vi "3_Analog_Meter_Reader(Inference).vi"() -> ()   [LabVIEW 2020]
uses:
  <vilib>/Ngene/DeepLTK/Toolkit/NN_Network/Controls/NN_Save_Before_Destroy_Options.ctl
  <vilib>/Ngene/DeepLTK/Toolkit/NN_Layers/Layers/Input/API/NN_Layer_Set_Out(Input3D_idx).vi
  <vilib>/Ngene/DeepLTK/Toolkit/Deep_Learning_Toolkit_by_Ngene.lvlib
  <vilib>/vision/NI_Vision_Development_Module.lvlib
panel:
  out "Inference Speed (FPS)":dbl=427.1678770791453
  out "Image Path":path=path "D:/DeepLTK_Examples/Analog_Meter/Train/Images/0537.png"
  in  "Stop":bool
  out "Predictions":sgl[](array[slide])=[74.73664] scale=0.0..10.0
  in  "mBatch":i32=1
  in  "NN Device":enum16{"CPU", "GPU"}(ring)=enum."GPU"
  in  "Network Configuration File Path":path=path "D:/Ngene/GitHub/deepltk_examples/3_Image_Processing/31_Image_Regression/working/Analog_Meter/Analog_Meter_net_cfg_23_11_29__18_30_17.cfg"
  in  "Weight File Path":path=path "D:/Ngene/GitHub/deepltk_examples/3_Image_Processing/31_Image_Regression/working/Analog_Meter/Analog_Meter_weights_23_11_29__18_30_17.bin"
  in  "File Path":path=path "D:/DeepLTK_Examples/Analog_Meter/Train/Images/0537.png"
  out "Image":T1(plugin-control)
  # "Instructions:\n1. Provide model files (.cfg and .bin).\n2. Run the VI\n3. Drag and drop image on \"Input Image\"\n4. Observe rge prediction result."
  # "Input Image"
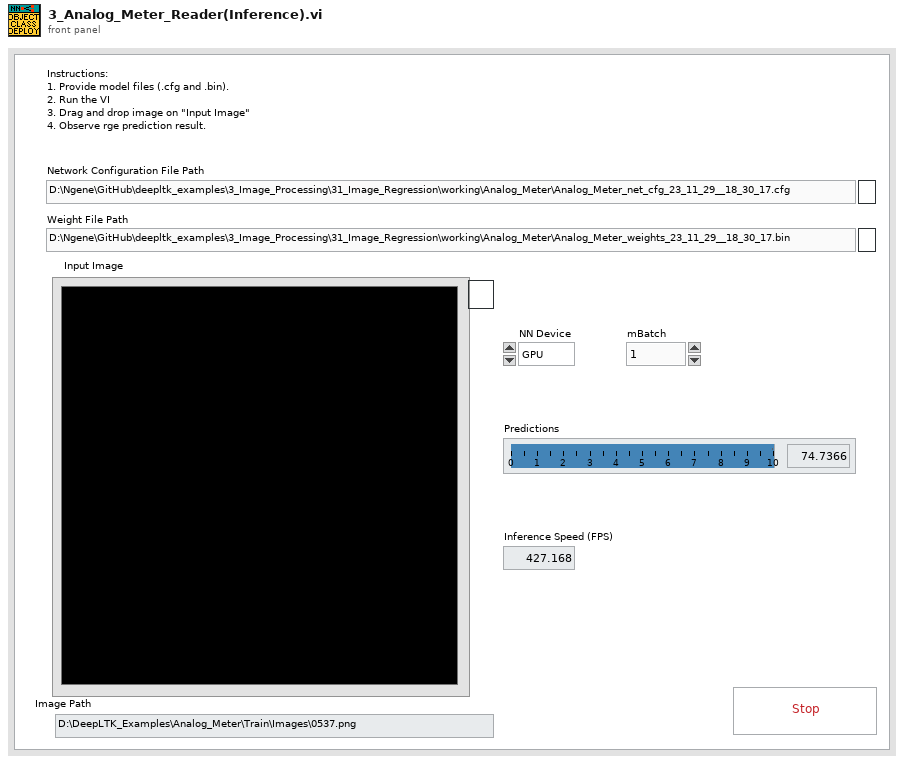
[diagram p1: front panel]
types:
  T1 = typedef "IMAQ Image.ctl" = refnum<image>
  T2 = typedef "Image Type" = u32
  T3 = typedef "Deep_Learning_Toolkit_by_Ngene.lvlib/NN_Save_Before_Destroy_Options.ctl" = cluster{"CFG?":bool, "Weights?":bool, "Render?":bool}
  T4 = typedef "Deep_Learning_Toolkit_by_Ngene.lvlib/NN_Config_Params.ctl" = cluster{"Name":string, "mBatch":i32, "NN_Train_Params":T5, "LR_Decay_Policy":T8, "Labels":string[], "Loss":T10}
  T5 = typedef "Deep_Learning_Toolkit_by_Ngene.lvlib/NN_Train_Params.ctl" = cluster{"Optimizer":T6, "Beta_1":sgl, "Beta_2":sgl, "Weight Decay(L1)":sgl, "Weight Decay(L2)":sgl, "Data_Sampling":T7}
  T6 = typedef "Deep_Learning_Toolkit_by_Ngene.lvlib/NN_Train_Optimizer.ctl" = enum16{"SGD", "Adam", "Adagrad", "Adadelta", "RMSProp", "Nesterov"}
  T7 = typedef "Deep_Learning_Toolkit_by_Ngene.lvlib/NN_Train_Data_Sampling.ctl" = enum16{"Random", "Sequential"}
  T8 = typedef "Deep_Learning_Toolkit_by_Ngene.lvlib/NN_LR_Policy_Cfg.ctl" = cluster{"Policy_Type":T9, "LR0":dbl, "k":sgl, "WarmUp_Policy":enum16{"Step", "Ramp"}, "WarmUp_Iter":i32, "WarmUp_Ratio":sgl}
  T9 = typedef "Deep_Learning_Toolkit_by_Ngene.lvlib/NN_LR_Policy_Type.ctl" = enum16{"Manual", "Step", "Exp", "1/t"}
  T10 = typedef "Deep_Learning_Toolkit_by_Ngene.lvlib/NN_Loss_Config_Params.ctl" = cluster{"Loss_Type":T11, "Loss_Conf_Params":variant}
  T11 = typedef "Deep_Learning_Toolkit_by_Ngene.lvlib/NN_Loss_Type.ctl" = enum16{"None", "MSE", "CrossEntropy", "YOLO_v2"}
  T12 = typedef "Deep_Learning_Toolkit_by_Ngene.lvlib/NN_Layer_Config_Params.ctl" = cluster{"Layer_Type":T13, "Layer_Conf_Params":variant}
  T13 = typedef "Deep_Learning_Toolkit_by_Ngene.lvlib/NN_Layer_Type.ctl" = enum16{"Input1D", "Input3D", "Conv2D", "Conv2D_Adv", "MaxPool", "AvgPool", "UpSample", "DropOut3D", "ShortCut", "Concat", "SoftMax3D", "FC", "DropOut", "Softmax", "Flatten", "YOLO_v2", "Unsupported"}
  T14 = typedef "Deep_Learning_Toolkit_by_Ngene.lvlib/NN.ctl" = cluster{"Name":string, "No of Layers":i32, "mBatch":i32, "Layers":T15[], "Dimty":T16, "Dims_In":T17, "Dims_Out":T17, "Working_Dir":path, "Train?":bool, "Train_Params":T5, "LR_Update_Policy":T8, "Session Data":T18, "Ground_truth":T19, "NNg_hdls":T21, "NN_Device":T22, "GPU Id":i32, "Labels":string[], "Receptive Field":T23[], "Loss_Type":T11, "Loss_Cfg_Prms":variant}
  T15 = typedef "Deep_Learning_Toolkit_by_Ngene.lvlib/NN_Layer_ref.ctl" = refnum<data-value>
  T16 = typedef "Deep_Learning_Toolkit_by_Ngene.lvlib/NN_In_Out_Dim-ty.ctl" = enum8{"In1D_Out1D", "In3D_Out1D", "In3D_Out3D", "In3D_OutBBox"}
  T17 = typedef "Deep_Learning_Toolkit_by_Ngene.lvlib/NN_Dims(C,H,W).ctl" = cluster{"C":i32, "H":i32, "W":i32}
  T18 = typedef "Deep_Learning_Toolkit_by_Ngene.lvlib/NN_Train_Session_Data.ctl" = cluster{"Epochs":sgl, "Tot_Iter":i32, "LR":sgl, "LR_iter":i32}
  T19 = typedef "Deep_Learning_Toolkit_by_Ngene.lvlib/NN_Ground_truth.ctl" = cluster{"Y":variant, "Y_idx":T20}
  T20 = typedef "Deep_Learning_Toolkit_by_Ngene.lvlib/NN_Data_ref(1D_I32).ctl" = refnum<data-value>
  T21 = typedef "Deep_Learning_Toolkit_by_Ngene.lvlib/nng_cuda_handles.ctl" = cluster{"cudnn":u64, "cublas":u64, "stream":u64, "curand":u64}
  T22 = typedef "Deep_Learning_Toolkit_by_Ngene.lvlib/NN_Device.ctl" = enum16{"CPU", "GPU"}
  T23 = typedef "Deep_Learning_Toolkit_by_Ngene.lvlib/NN_Dims(V,H).ctl" = cluster{"V":i32, "H":i32}
  T24 = typedef "Deep_Learning_Toolkit_by_Ngene.lvlib/NN_Layer.ctl" = cluster{"Name":string, "Layer_Data":variant, "Layer_Type":T13, "Dims_In":T17, "Layers_In":variant, "Dims_Out":T17, "Layers_Out":variant, "Metrics":T25, "GPU_Data":variant, "mBatch":i32, "NN_Device":T22, "NNg_hdls":T21, "Train?":bool, "Dimty":T26, "RecptField":T27}
  T25 = typedef "Deep_Learning_Toolkit_by_Ngene.lvlib/NN_Layer_Metrics.ctl" = cluster{"Data":dbl, "Params":dbl, "Ops":dbl}
  T26 = typedef "Deep_Learning_Toolkit_by_Ngene.lvlib/NN_Layer_Dimty.ctl" = enum16{"1D", "3D"}
  T27 = typedef "Deep_Learning_Toolkit_by_Ngene.lvlib/NN_Layer_RF_State.ctl" = cluster{"Dims":T23, "J":T23}
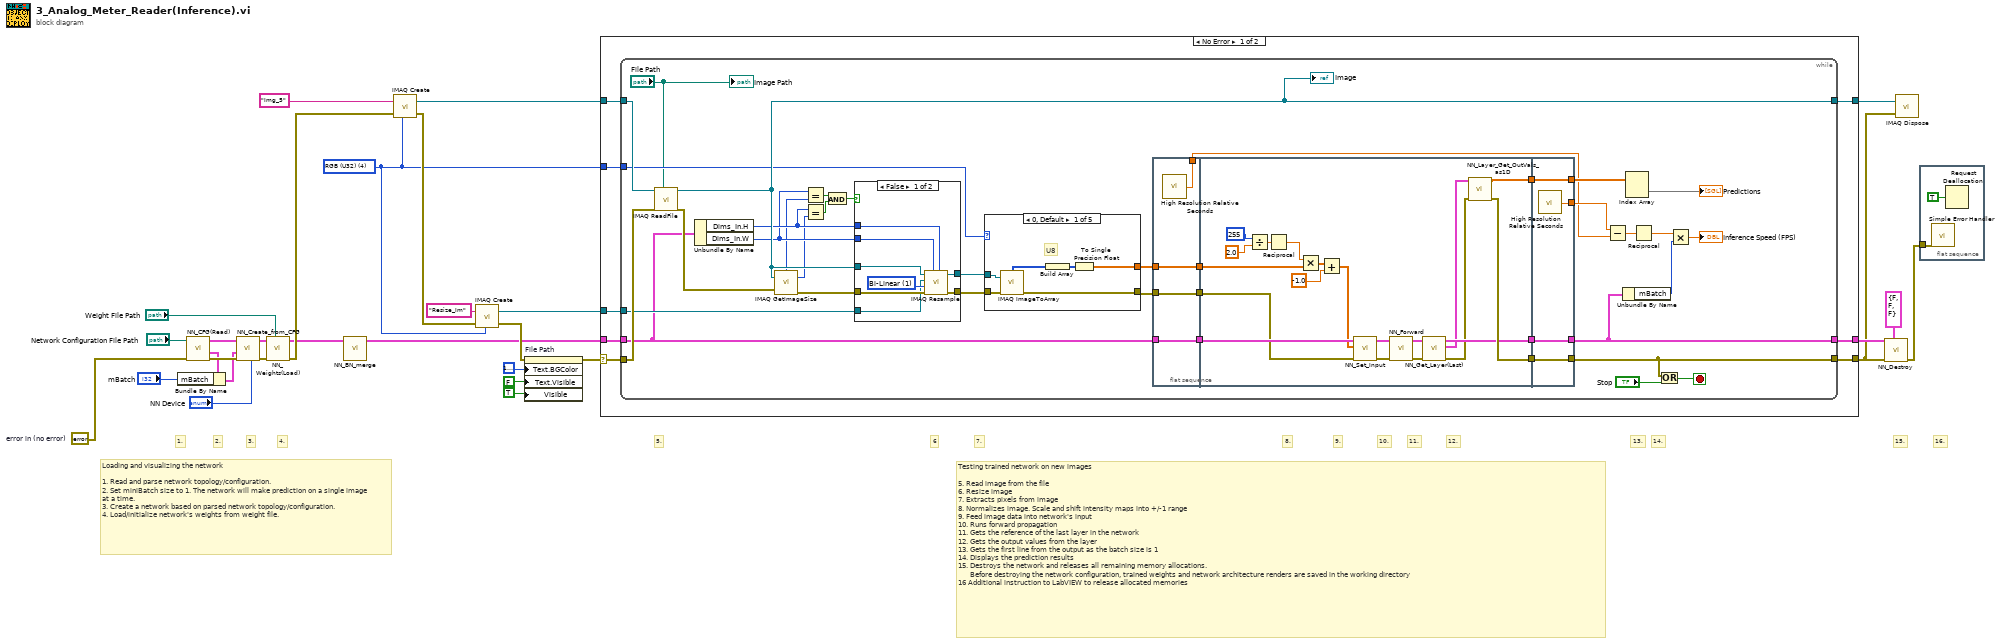
[diagram p0: block diagram]
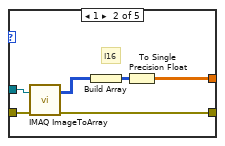
[diagram p3: hidden frame]
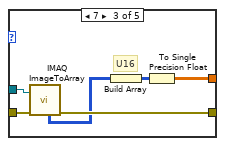
[diagram p4: hidden frame]
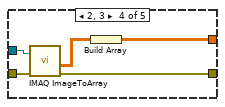
[diagram p5: hidden frame]
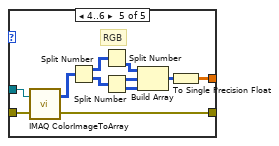
[diagram p6: hidden frame]
diagram:
  w2 = T2 4 items=["Grayscale (U8)", "Grayscale (I16)", "Grayscale (SGL)", "Complex (CSG)", "RGB (U32)", "HSL (U32)", "RGB (U64)", "Grayscale (U16)"] ("Image Type")
  w8 = errorcluster {"status"=FALSE, "code"=0, "source"=""}  # error in (no error)
  # "6"
  # "Testing trained network on new images\n\n5. Read image from the file\n6. Resize image\n7. Extracts pixels from image\n8. Normalizes image. Scale and shift intensity maps into +/-1 range\n9. Feed image data into network's input\n10. Runs forward propagation\n11. Gets the reference of the last layer in the network\n12. Gets the output values from the layer\n13. Gets the first line from the output as the batch size is 1\n14. Displays the prediction results\n15. Destroys the network and releases all remaining memory allocations.\n      Before destroying the network configuration, trained weights and network architecture renders are saved in the working directory\n16 Additional instruction to LabVIEW to release allocated memories"
  # "16."
  # "15."
  # "14."
  # "Loading and visualizing the network\n\n1. Read and parse network topology/configuration.\n2. Set miniBatch size to 1. The network will make prediction on a single image at a time.\n3. Create a network based on parsed network topology/configuration.\n4. Load/initialize network's weights from weight file."
  # "4."
  # "3."
  # "2."
  # "1."
  # "13."
  # "12."
  # "11."
  # "10."
  # "9."
  # "8."
  # "7."
  # "5."
  n1 = call <vilib>:"NN_CFG(Read).vi"("error in (no error)"=w8, "CFG file path"="Network Configuration File Path") -> ("error out"=w29:errorcluster, "Net_Cfg"=w15:T4, "Layer_Cfg"=w14:T12[])  [unwired: 7 in]
  n2 = Bundle By Name(cluster=w15, "mBatch"="mBatch") -> (w10:T4)
  n3 = call <vilib>:"NN_Create_from_CFG.vi"("NN_Device"="NN Device", "error in (no error)"=w29, "Net_Cfg"=w10, "Layer_Cfg"=w14) -> ("error out"=w17:errorcluster, "NN out"=w13:T14)  [unwired: 6 in]
  n4 = call <vilib>:"NN_Weights(Load).vi"("Weight File Path"="Weight File Path", "error in (no error)"=w17, "NN in"=w13) -> ("error out"=w30:errorcluster, "NN out"=w12:T14)  [unwired: 7 in]
  n5 = call <vilib>:"NN_BN_merge.vi"("NN in"=w12) -> ("NN out"=w1:T14)  [unwired: 9 in, 1 out]
  n6 = call "IMAQ Create"("Image Name"="Img_5", "Image Type"=w2, "error in (no error)"=w30) -> ("New Image"=w19:T1, "error out"=w6:errorcluster)  [unwired: 2 in]
  n7 = call "IMAQ Create"("Image Name"="Resize_Im", "Image Type"=w2, "error in (no error)"=w6) -> ("New Image"=w4:T1, "error out"=w5:errorcluster)  [unwired: 2 in]
  n8 = property on="File Path" class="Path"(error in=w5, "Text.BGColor"=u32 16777216, "Text.Visible"=FALSE ("Path Text.Visible"), "Visible"=TRUE) -> (error out=w11:errorcluster)  [unwired: 1 in, 1 out]
  n9 = case shown="No Error" w11 {
    selector: w11 -> [w34 w148]
    tunnel: w1 -> [w38 w149]
    tunnel: [w37 w149] -> w21
    tunnel: [w36 w148] -> w20
    tunnel: [w35 w150] -> w22
    tunnel: w19 -> [w33 w150]
    tunnel: w2 -> [w32 _]
    tunnel: w4 -> [w31 _]
    frame No Error {
      n10 = while {
        tunnel: w34 -> [w76]
        tunnel: w38 -> [w68]
        tunnel: [w63] -> w37
        tunnel: [w64] -> w36
        tunnel: [w71] -> w35
        tunnel: w33 -> [w75]
        tunnel: w32 -> [w70]
        tunnel: w31 -> [w69]
        stop <- w65 stop-if-true
        n11 = call "IMAQ ReadFile"("File Path"="File Path", "error in (no error)"=w76, "Image"=w75) -> ("error out"=w73:errorcluster, "Image Out"=w71:T1)  [unwired: 4 in, 3 out]
        "Image" <- w71
        n12 = Unbundle By Name(w68) -> ("Dims_In.H"=w67:i32, "Dims_In.W"=w66:i32)
        n13 = call "IMAQ GetImageSize"("Image"=w71, "error in (no error)"=w73) -> ("Y Resolution"=w58:i32, "X Resolution"=w59:i32, "error out"=w57:errorcluster)  [unwired: 2 in]
        n14 = Equal?(x=w66, y=w59) -> (x = y?=w61:bool)
        n15 = Equal?(x=w67, y=w58) -> (x = y?=w60:bool)
        n16 = And(x=w61, y=w60) -> (x .and. y?=w56:bool)
        n17 = case shown="False" w56 {
          tunnel: [w111 w113] -> w54
          tunnel: w71 -> [w105 w113]
          tunnel: [w110 w112] -> w55
          tunnel: w67 -> [w109 _]
          tunnel: w57 -> [w107 w112]
          tunnel: w66 -> [w106 _]
          tunnel: w69 -> [w104 _]
          frame False {
            w108 = u32 1 items=["Zero Order", "Bi-Linear", "Quadratic", "Cubic Spline"] ("Interpolation Type")
            n18 = call "IMAQ Resample"("X Resolution"=w109, "Y Resolution"=w106, "error in (no error)"=w107, "Interpolation Type"=w108, "Image Dst"=w104, "Image Src"=w105) -> ("error out"=w110:errorcluster, "Image Dst Out"=w111:T1)  [unwired: 4 in]
          }
          frame True {
          }
        }
        n19 = case shown="0, Default" w70 {
          tunnel: w54 -> [w115 w122 w128 w134 w141]
          tunnel: w55 -> [w119 w125 w131 w136 w147]
          tunnel: [w117 w124 w130 w135 w145] -> w52
          tunnel: [w114 w121 w127 w133 w137] -> w53
          frame 0, Default {
            # "U8"
            n20 = call "IMAQ ImageToArray"("error in (no error)"=w119, "Image"=w115) -> ("error out"=w117:errorcluster, "Image Pixels (U8)"=w118:u8[][])  [unwired: 2 in, 3 out]
            n21 = Build Array(w118) -> (w116:u8[][][])
            n22 = To Single Precision Float(number=w116) -> (single precision float=w114:sgl[][][])
          }
          frame 1 {
            # "I16"
            n23 = call "IMAQ ImageToArray"("error in (no error)"=w125, "Image"=w122) -> ("error out"=w124:errorcluster, "Image Pixels (I16)"=w120:i16[][])  [unwired: 2 in, 3 out]
            n24 = Build Array(w120) -> (w123:i16[][][])
            n25 = To Single Precision Float(number=w123) -> (single precision float=w121:sgl[][][])
          }
          frame 7 {
            # "U16"
            n26 = call "IMAQ ImageToArray"("error in (no error)"=w131, "Image"=w128) -> ("Image Pixels (U16)"=w126:u16[][], "error out"=w130:errorcluster)  [unwired: 2 in, 3 out]
            n27 = Build Array(w126) -> (w129:u16[][][])
            n28 = To Single Precision Float(number=w129) -> (single precision float=w127:sgl[][][])
          }
          frame 2, 3 {
            n29 = call "IMAQ ImageToArray"("error in (no error)"=w136, "Image"=w134) -> ("Image Pixels (Float)"=w132:sgl[][], "error out"=w135:errorcluster)  [unwired: 2 in, 3 out]
            n30 = Build Array(w132) -> (w133:sgl[][][])
          }
          frame 4..6 {
            # "RGB"
            n31 = call "IMAQ ColorImageToArray"("Image"=w141, "error in (no error)"=w147) -> ("Image Pixels (U32)"=w146:u32[][], "error out"=w145:errorcluster)  [unwired: 2 in, 1 out]
            n32 = Split Number(x=w146) -> (hi(x)=w143:u16[][], lo(x)=w144:u16[][])
            n33 = Split Number(x=w143) -> (lo(x)=w140:u8[][])  [unwired: 1 out]
            n34 = Split Number(x=w144) -> (hi(x)=w139:u8[][], lo(x)=w138:u8[][])
            n35 = Build Array(w140, w139, w138) -> (w142:u8[][][])
            n36 = To Single Precision Float(number=w142) -> (single precision float=w137:sgl[][][])
          }
        }
        n37 = flat-sequence {
          tunnel: w52 -> [w78]
          tunnel: w53 -> [w79]
          tunnel: w68 -> [w80]
          tunnel: [w80] -> w51
          tunnel: [w79] -> w50
          tunnel: [w78] -> w49
          tunnel: [w77] -> w44
          tunnel: w51 -> [w98]
          tunnel: w50 -> [w83]
          tunnel: w49 -> [w82]
          tunnel: [w99] -> w48
          tunnel: [w97] -> w47
          tunnel: [w96] -> w46
          tunnel: [w101] -> w63
          tunnel: [w102] -> w64
          tunnel: [w103] -> w74
          tunnel: w48 -> [w103]
          tunnel: w47 -> [w102]
          tunnel: w46 -> [w101]
          tunnel: [w100] -> w45
          frame #0 {
            n38 = call <vilib>:"High Resolution Relative Seconds.vi"() -> ("relative seconds"=w77:dbl)
          }
          frame #1 {
            n39 = Divide(x=u16 255 ("dimension size"), y=sgl 2.0 ("dimension size")) -> (x/y=w85:sgl)
            n40 = Reciprocal(x=w85) -> (1/x=w81:sgl)
            n41 = Multiply(x=w81, y=w83) -> (x*y=w93:sgl[][][])
            n42 = Add(x=w93, y=sgl -1.0 ("dimension size")) -> (x+y=w92:sgl[][][])
            n43 = call-poly <vilib>:"NN_Set_Input.vi"("error in (no error)"=w82, "Data_In(3D_SGL)"=w92, "NN in"=w98) -> ("error out"=w90:errorcluster, "NN out"=w89:T14)  [unwired: 7 in]
            n44 = call <vilib>:"NN_Forward.vi"("error in (no error)"=w90, "NN in"=w89) -> ("error out"=w88:errorcluster, "NN out"=w87:T14)  [unwired: 6 in, 2 out]
            n45 = call <vilib>:"NN_Get_Layer(Last).vi"("error in (no error)"=w88, "NN in"=w87) -> ("error out"=w95:errorcluster, "Last_Layer"=w91:T24, "NN out"=w96:T14)  [unwired: 6 in, 1 out]
            n46 = call <vilib>:"NN_Layer_Get_OutVals_as1D.vi"("error in (no error)"=w95, "Layer"=w91) -> ("error out"=w97:errorcluster, "Out(as1D)"=w99:sgl[][])  [unwired: 8 in]
          }
          frame #2 {
            n47 = call <vilib>:"High Resolution Relative Seconds.vi"() -> ("relative seconds"=w100:dbl)
          }
        }
        n48 = Subtract(x=w45, y=w44) -> (x-y=w39:dbl)
        n49 = Unbundle By Name(w63) -> ("mBatch"=w62:i32)
        n50 = Index Array(array=w74) -> (element=→"Predictions":sgl[])  [unwired: 2 in]
        n51 = Reciprocal(x=w39) -> (1/x=w72:dbl)
        n52 = Or(x=w64, y="Stop") -> (x .or. y?=w65:bool)
        n53 = Multiply(x=w72, y=w62) -> (x*y=→"Inference Speed (FPS)":dbl)
        "Image Path" <- "File Path"
      }
    }
    frame Error {
    }
  }
  n54 = call <vilib>:"NN_Destroy.vi"("Save (T, T, T)"=T3 {"CFG?"=FALSE, "Weights?"=FALSE, "Render?"=FALSE} ("Save_Config"), "error in (no error)"=w20, "NN in"=w21) -> ("error out"=w23:errorcluster)  [unwired: 8 in]
  n55 = call "IMAQ Dispose"("Image"=w22, "error in (no error)"=w20) -> ()  [unwired: 4 in, 1 out]
  n56 = flat-sequence {
    tunnel: w23 -> [w152]
    frame #0 {
      n57 = call <vilib>:"Simple Error Handler.vi"("error in (no error)"=w152) -> ()  [unwired: 4 in, 5 out]
      n58 = Request Deallocation(TRUE ("flag")) -> ()
    }
  }
